vi "convert seconds to timespec.vi"(11 "seconds":dbl format="%#.6f") -> (3 "timespec":T1)   [LabVIEW 2013, in "Linux RT Utilities.lvlib"]
uses:
  Linux RT Utilities.lvlib
  Controls/Public/C Structs/timespec_64.ctl
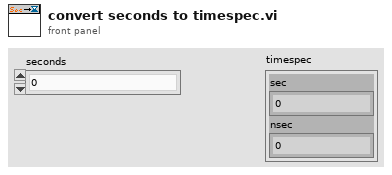
[diagram p1: front panel]
types:
  T1 = typedef "Linux RT Utilities.lvlib/timespec_64.ctl" = cluster{"sec":u64, "nsec":u64}
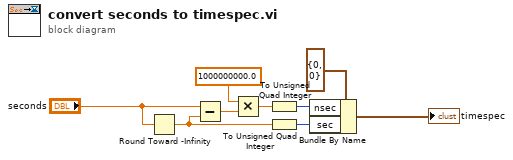
[diagram p0: block diagram]
diagram:
  n1 = Round Toward -Infinity(1:"seconds") -> (0:w1:dbl)
  n2 = Subtract(x="seconds", y=w1) -> (x-y=w5:dbl)
  n3 = Multiply(x=1000000000.0 ("y"), y=w5) -> (x*y=w6:dbl)
  n4 = To Unsigned Quad Integer(1:w6) -> (0:w3:u64)
  n5 = To Unsigned Quad Integer(1:w1) -> (0:w2:u64)
  n6 = Bundle By Name(cluster=T1 {"sec"=0, "nsec"=0} ("timespec"), "nsec"=w3, "sec"=w2) -> (→"timespec":T1)
